vi "DVR Update Connected.vi"(8 "error in (no error)":errorcluster, 10 "Connected":bool, 11 "Model_AMC in":refnum<class "Model_AMC.lvclass">) -> (0 "error out":errorcluster, 3 "Model_AMC out":refnum<class "Model_AMC.lvclass">)   [LabVIEW 2021, in "Model_AMC.lvclass"]
uses:
  Model_AMC.lvclass
  Model_AMC.lvclass/Model_AMC.ctl
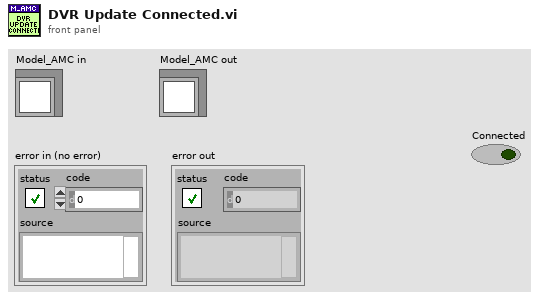
[diagram p1: front panel]
types:
  T1 = typedef "Model_AMC.lvclass/DVR.ctl" = cluster{"JKI_Network_Streams":refnum<class "NetworkConnection.lvclass">, "AMC Q":T2, "Connnected":bool}
  T2 = typedef "Model_AMC.lvclass/AMC Q.ctl" = cluster{"Main":T3, "OPCUA":T3, "NetworkSteam":T3}
  T3 = typedef "AMC_FW.lvlib/Queue.ctl" = cluster{"Q":T4, "Name":string}
  T4 = typedef "AMC_FW.lvlib/Message Queue.ctl" = refnum<queue>
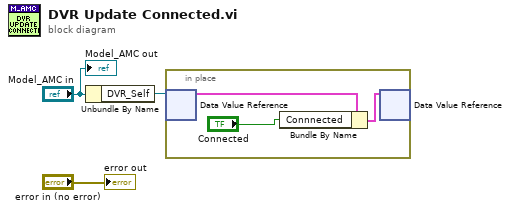
[diagram p0: block diagram]
diagram:
  n1 = Unbundle By Name("Model_AMC in") -> ("DVR_Self"=w2:refnum<data-value>)
  n2 = in-place {
    n3 = in-place-dvr #1(w2) -> (w6:T1)  [unwired: 1 out]
    n4 = Bundle By Name(cluster=w6, "Connnected"="Connected") -> (w5:T1)
    n5 = in-place-dvr #1(w5) -> ()  [unwired: 2 out]
  }
  "error out" <- "error in (no error)"
  "Model_AMC out" <- "Model_AMC in"
